vi "The library at a glance (README).vi"   [LabVIEW 2018, in "text_file.lvlib"]
uses:
  text_file.lvlib
  private_data (library_variable).vi
panel:
  # "The library at a glance"
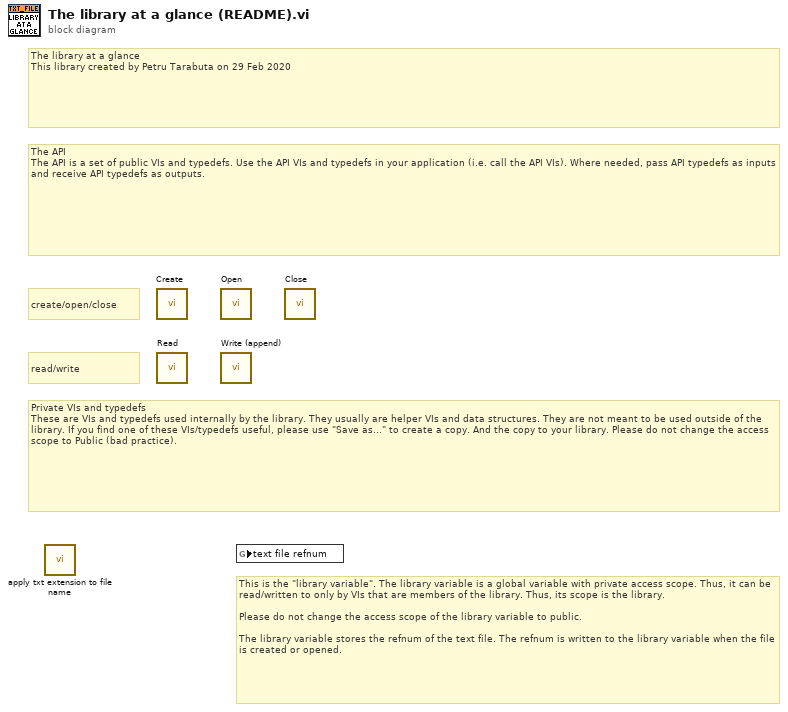
[diagram p0: block diagram]
diagram:
  # "This is the \"library variable\". The library variable is a global variable with private access scope. Thus, it can be read/written to only by VIs that are members of the library. Thus, its scope is the library.\n\nPlease do not change the access scope of the library variable to public.\n\nThe library variable stores the refnum of the text file. The refnum is written to the library variable when the file is created or opened."
  # "Private VIs and typedefs\nThese are VIs and typedefs used internally by the library. They usually are helper VIs and data structures. They are not meant to be used outside of the library. If you find one of these VIs/typedefs useful, please use \"Save as...\" to create a copy. And the copy to your library. Please do not change the access scope to Public (bad practice)."
  # "read/write"
  # "create/open/close"
  # "The API\nThe API is a set of public VIs and typedefs. Use the API VIs and typedefs in your application (i.e. call the API VIs). Where needed, pass API typedefs as inputs and receive API typedefs as outputs."
  # "The library at a glance\nThis library created by Petru Tarabuta on 29 Feb 2020"
  n1 = call "apply txt extension to file name.vi"() -> ()  [unwired: 1 in, 1 out]
  n2 = call "Create.vi"() -> ()  [unwired: 10 in, 2 out]
  n3 = call "Read.vi"() -> ()  [unwired: 11 in, 1 out]
  n4 = call "Open.vi"() -> ()  [unwired: 11 in, 1 out]
  n5 = call "Write (append).vi"() -> ()  [unwired: 11 in, 1 out]
  n6 = global read "private_data (library_variable).vi" "text file refnum"() -> ()  [unwired: 1 in]
  n7 = call "Close.vi"() -> ()  [unwired: 11 in, 1 out]
